vi "TestingEnvironment.vi"() -> ()   [LabVIEW 2023]
panel:
  out "Waveform Chart":T1(graph)
  out "String":string
  out "Array":dbl[](array[numeric])
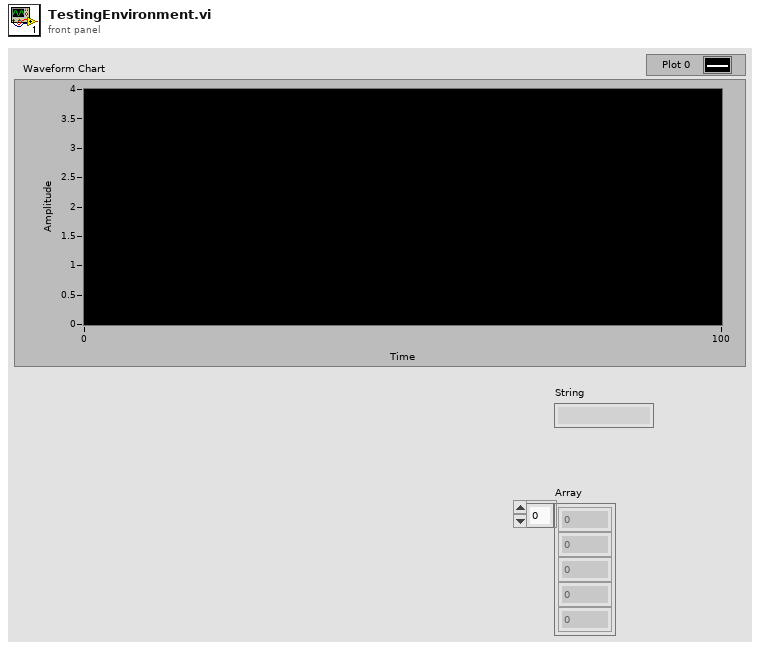
[diagram p1: front panel]
types:
  T1 = cluster{"array type (2D Dbl)[0]":dbl, "array type (2D Dbl)[1]":dbl, "array type (2D Dbl)[2]":dbl, "array type (2D Dbl)[3]":dbl, "array type (2D Dbl)[4]":dbl, "array type (2D Dbl)[5]":dbl, "array type (2D Dbl)[6]":dbl, "array type (2D Dbl)[7]":dbl, "array type (2D Dbl)[8]":dbl}
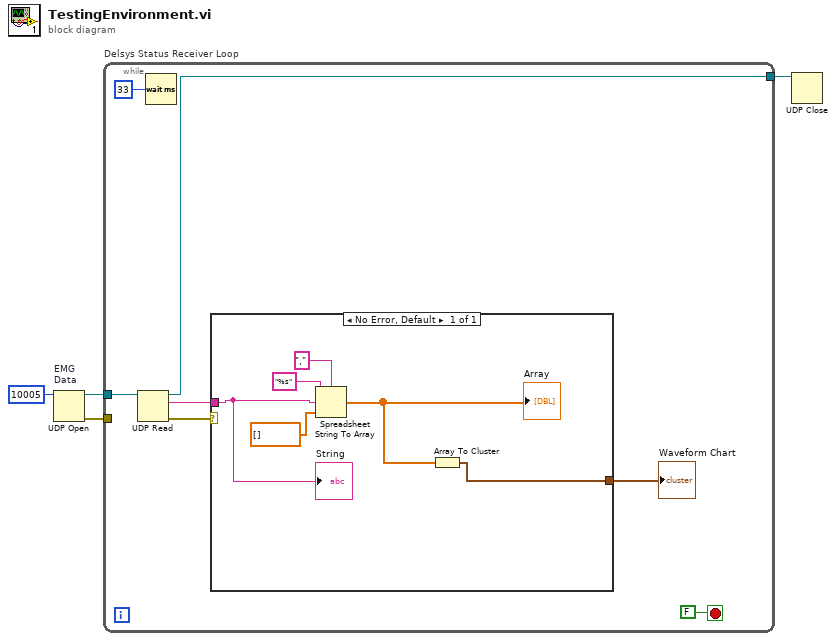
[diagram p0: block diagram]
diagram:
  n1 = UDP Open "EMG\nData"(11:u16 10005 ("port")) -> (port=w1:refnum<k16>, 0:w2:errorcluster)  [unwired: 4 in, 1 out]
  n2 = while "Delsys Status Receiver Loop" {
    tunnel: [w6] -> w4
    tunnel: w2 -> [_]
    tunnel: w1 -> [w9]
    stop <- FALSE stop-if-true
    n3 = UDP Read(connection ID=w9) -> (data out=w7:string, error out=w8:errorcluster, 3:w6:refnum<k16>)  [unwired: 3 in, 2 out]
    n4 = Wait (ms)(milliseconds to wait=33) -> ()  [unwired: 1 out]
    n5 = case shown="No Error, Default" w8 {
      tunnel: w7 -> [w14]
      tunnel: [w12] -> w5
      frame No Error {
        n6 = Spreadsheet String To Array(delimiter (Tab)=",", format string="%s", spreadsheet string=w14, array type (2D Dbl)=dbl[] []) -> (array=w13:dbl[])
        "Array" <- w13
        n7 = Array To Cluster(array=w13) -> (cluster=w12:T1)
        "String" <- w14
      }
    }
    "Waveform Chart" <- w5
  }
  n8 = UDP Close(connection ID=w4) -> ()  [unwired: 1 in, 2 out]
